vi "Start Measurement.vi"(8 "error in (no error)":errorcluster, 10 "Launch Measurements Message in":refnum<class "Launch Measurements Message.lvclass">, 11 "Client Controller in":refnum<class "Client Controller.lvclass">) -> (0 "error out":errorcluster, 3 "Client Controller out":refnum<class "Client Controller.lvclass">)   [LabVIEW 2026, in "Client Controller.lvlib" / "Client Controller.lvclass"]
uses:
  Client Controller.lvclass
  C:/Users/E2013170/Documents/GitHub/Measurement-Utility-Reference/components/MAL-Framework/user.lib/Common Components/Controller/Controller.lvclass
  MAL-Framework/user.lib/Common Components/Controller/Messages/Launch Measurements Message/Launch Measurements Message.lvclass
  MAL-Framework/user.lib/Common Components/Controller/Messages/Launch Measurements Message/Launch Measurements Message.lvclass/Launch Measurements Message.ctl
  MAL-Framework/user.lib/Common Components/Controller/Controller.lvclass
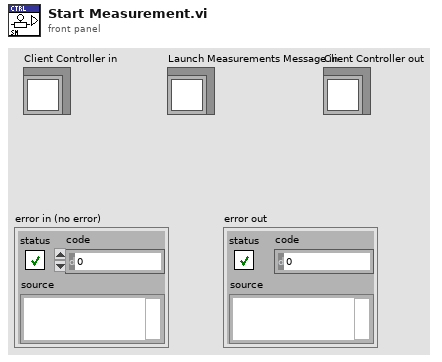
[diagram p1: front panel]
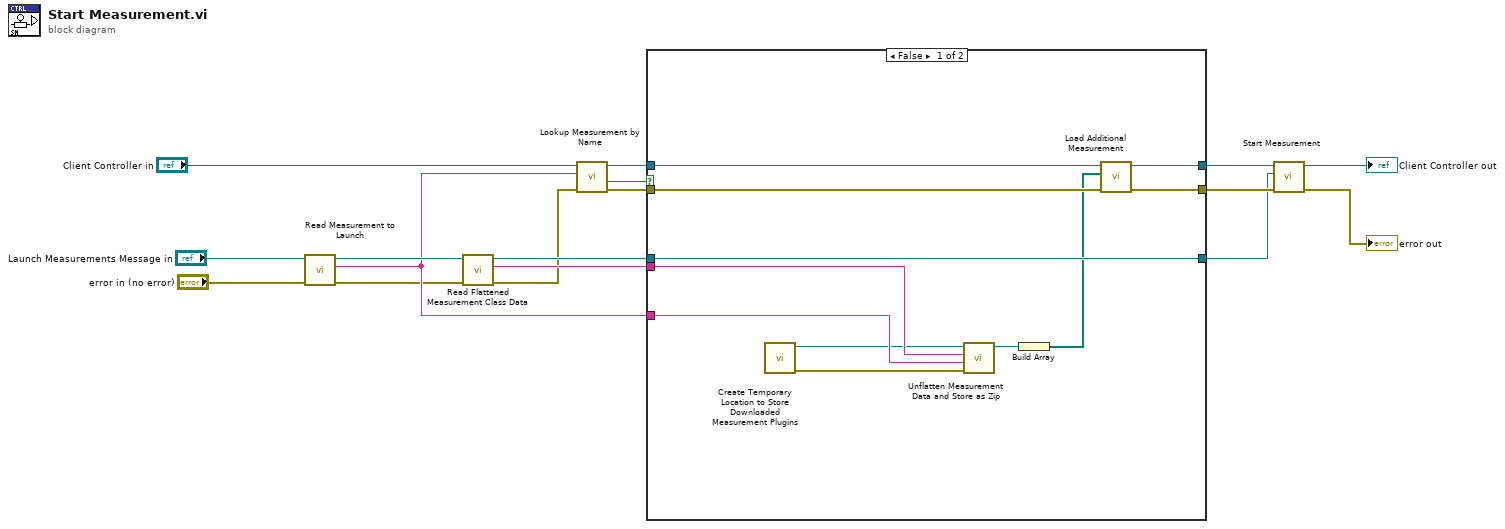
[diagram p0: block diagram]
diagram:
  n1 = call "Read Measurement to Launch.vi"("error in (no error)"="error in (no error)", "Launch Measurements Message in"="Launch Measurements Message in") -> ("error out"=w2:errorcluster, "Measurement Name"=w8:string, "Launch Measurements Message out"=w10:refnum<class "Launch Measurements Message.lvclass">)  [unwired: 7 in]
  n2 = call "Read Flattened Measurement Class Data.vi"("error in (no error)"=w2, "Launch Measurements Message in"=w10) -> ("error out"=w3:errorcluster, "Flattened Measurement Class Data"=w4:string, "Launch Measurements Message out"=w6:refnum<class "Launch Measurements Message.lvclass">)  [unwired: 7 in]
  n3 = call "Lookup Measurement by Name.vi"("error in (no error)"=w3, "Measurement Name"=w8, "Controller in"="Client Controller in") -> ("error out"=w12:errorcluster, "found"=w15:bool, "Controller out"=w14:refnum<class "Client Controller.lvclass">)  [unwired: 5 in, 1 out]
  n4 = case shown="False" w15 {
    tunnel: w14 -> [w25 w31]
    tunnel: [w28 w31] -> w13
    tunnel: w8 -> [w26 _]
    tunnel: w12 -> [w24 w30]
    tunnel: [w27 w30] -> w11
    tunnel: w6 -> [w23 w29]
    tunnel: [w23 w29] -> w5
    tunnel: w4 -> [w22 _]
    frame False {
      n5 = call "Create Temporary Location to Store Downloaded Measurement Plugins.vi"() -> ("error out"=w21:errorcluster, "created path"=w18:path)  [unwired: 10 in]
      n6 = call "Unflatten Measurement Data and Store as Zip.vi"("error in (no error)"=w21, "Measurement Name"=w26, "Measurement Data"=w22, "Path to Store Measurement"=w18) -> ("Folder Location"=w20:path)  [unwired: 6 in, 1 out]
      n7 = Build Array(w20) -> (w19:path[])
      n8 = call "Load Additional Measurement.vi"("error in (no error)"=w24, "Array of Measurement Paths"=w19, "Controller in"=w25) -> ("error out"=w27:errorcluster, "Controller out"=w28:refnum<class "Client Controller.lvclass">)  [unwired: 7 in]
    }
    frame True {
    }
  }
  n9 = call-parent "Start Measurement.vi"("error in (no error)"=w11, "Launch Measurements Message in"=w5, "Controller in"=w13) -> ("error out"=→"error out":errorcluster, "Controller out"=→"Client Controller out":refnum<class "Client Controller.lvclass">)  [unwired: 7 in]
